vi "Scans.vi"(1 "Time zero (sec)":timestamp, 2 "Queue in":T1 {"Scan settings in queue" items=["Regular", "Inverted", "MartinaSettings"]; "Time of the last scan (s)" format="%<%H:%M:%S>t"; "When did you stick it in?" format="%<%H:%M:%S>t"; "Time to next scan (s)" format="%<%H:%M:%S>t"; "Time in rig (s)" format="%<%H:%M:%S>t"}) -> (0 "Queue out":T1 {"Scan settings in queue" items=["Regular", "Inverted", "MartinaSettings"]; "Time of the last scan (s)" format="%<%H:%M:%S>t"; "When did you stick it in?" format="%<%H:%M:%S>t"; "Time to next scan (s)" format="%<%H:%M:%S>t"; "Time in rig (s)" format="%<%H:%M:%S>t"})   [LabVIEW 2011]
uses:
  Typedefs/Queue.ctl
  Typedefs/Queue cluster.ctl
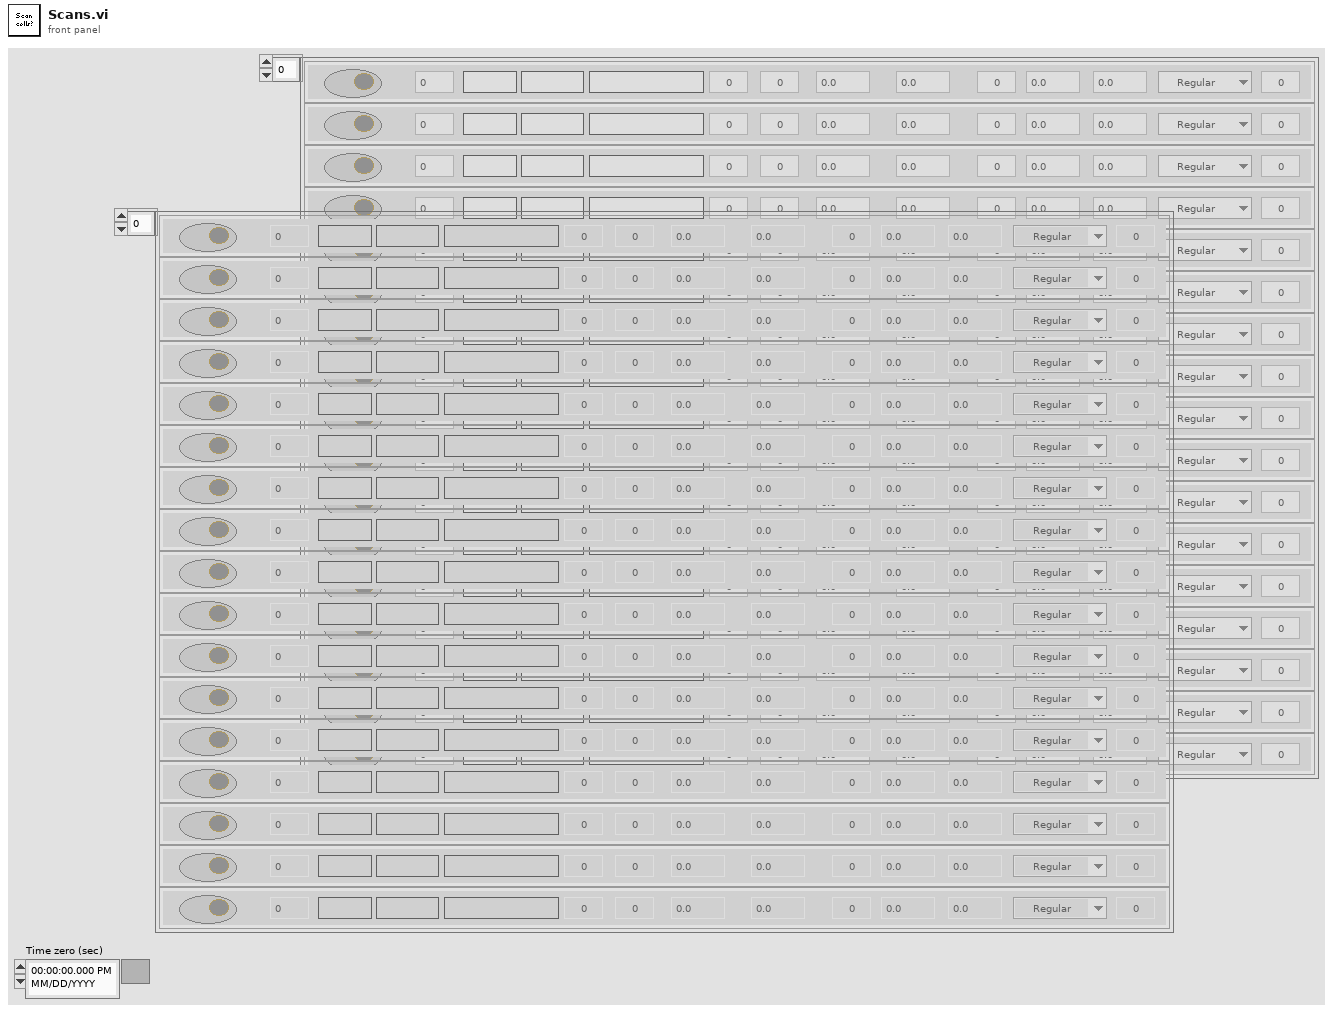
[diagram p1: front panel]
types:
  T1 = typedef "Queue.ctl" = T2[]
  T2 = typedef "Queue cluster.ctl" = cluster{"Measure?":bool, "Area (cm^2)":dbl, "Cell Label":string, "Cell Description":string, "Cell Position":i32, "Time in rig (s)":dbl, "Time to next scan (s)":dbl, "Scan number":dbl, "When did you stick it in?":dbl, "Time between scans (s)":dbl, "Time of the last scan (s)":dbl, "Scan settings in queue":u16, "Sample Holder":dbl, "User Name":string}
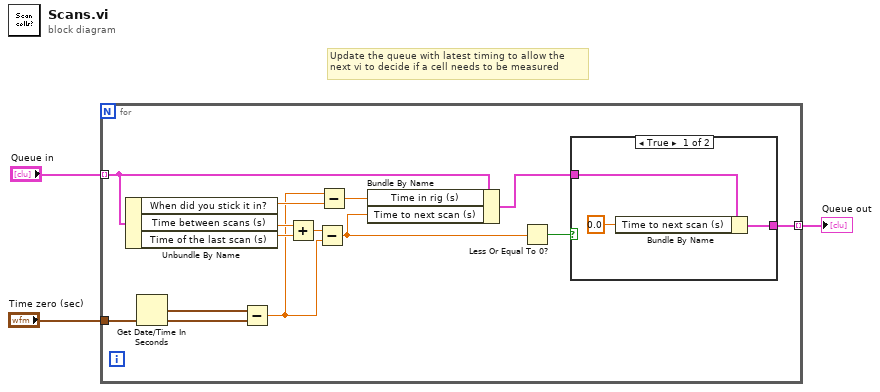
[diagram p0: block diagram]
diagram:
  # "Update the queue with latest timing to allow the \nnext vi to decide if a cell needs to be measured"
  n1 = for {
    tunnel: "Time zero (sec)" -> [w15]
    tunnel: "Queue in" -> [w12] mode=indexing
    tunnel: [w13] -> w1 mode=indexing
    n2 = Unbundle By Name(w12) -> ("When did you stick it in?"=w10:dbl, "Time between scans (s)"=w8:dbl, "Time of the last scan (s)"=w9:dbl)
    n3 = Get Date/Time In Seconds() -> (seconds since 1Jan1904=w16:timestamp)
    n4 = Subtract(x=w16, y=w15) -> (x-y=w6:dbl)
    n5 = Add(x=w8, y=w9) -> (x+y=w7:dbl)
    n6 = Subtract(x=w7, y=w6) -> (x-y=w4:dbl)
    n7 = Subtract(x=w6, y=w10) -> (x-y=w5:dbl)
    n8 = Bundle By Name(cluster=w12, "Time in rig (s)"=w5, "Time to next scan (s)"=w4) -> (w11:T2)
    n9 = Less Or Equal To 0?(x=w4) -> (x <= 0?=w14:bool)
    n10 = case shown="True" w14 {
      tunnel: w11 -> [w17 w20]
      tunnel: [w19 w20] -> w13
      frame True {
        n11 = Bundle By Name(cluster=w17, "Time to next scan (s)"=0.0 ("Time since last scan (min)")) -> (w19:T2)
      }
      frame False {
      }
    }
  }
  "Queue out" <- w1
